vi "Uframe-LVDT_Cal.vi"() -> ()   [LabVIEW 2010]
uses:
  <vilib>/Platform/TimedLoop/XDataNode/XDataNode.xnode
  <vilib>/Platform/TimedLoop/XDataNode/timing_clust.ctl
  <vilib>/Platform/TimedLoop/XDataNode/nitl_modes.ctl
  <vilib>/Platform/TimedLoop/XDataNode/wakeup.ctl
  <vilib>/Platform/TimedLoop/XDataNode/XDNodeRunTimeDep.lvlib
panel:
  out "Numeric":i32
  in  "Displacement (inch)":dbl min=-1.0 max=60.0 step=0.01
  in  "Begin":bool
  in  "Stop":bool
  out "Disp Vs Time":cluster{dbl[], dbl[]}(graph)={[-724.1250113144533, -724.195323815552, -724.2656363166506, -724.3359488177492, -724.4062613188479, -724.4765738199465, -724.5468863210451, -724.6171988221438, -724.7461050741579, -724.9218863269045, -725.0976675796511, -725.2851675825808, -725.4492300851442], [-11.89350874713131, -11.896152101474941, -11.894229661847117, -11.89350874707076, -11.890865392620372, -11.895671491596438, -11.895911796524977, -11.899756675680168, -11.899035760801853, -11.90552399441818, -11.907927043887174, -11.905283689458143, -11.914655582386047]}
  in  "File Name":string="Test"
  in  "File Path":path=path "C:/cygwin/home/Smarter Materials/Users 2010_2011/Chris_Montgomery"
  in  "Sample Notes":string
  in  "Data Acquisition Interval (s)":dbl min=0.01 max=60.0 step=0.01
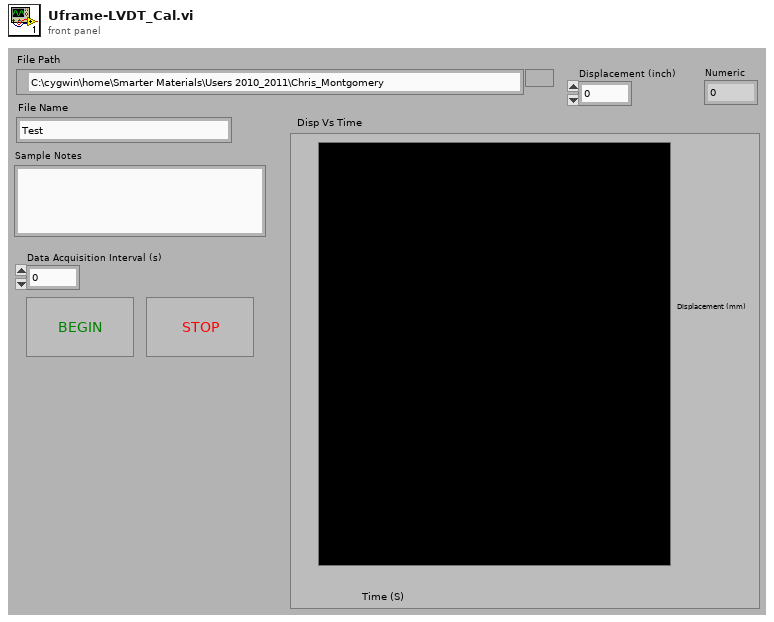
[diagram p1: front panel]
types:
  T1 = typedef "XDNodeRunTimeDep.lvlib/timing_clust.ctl" = cluster{"Expected End [f-1]":u64, "Actual End [f-1]":u64, "Finished Late? [f-1]":bool, "Expected End [i-1]":u64, "Actual End [i-1]":u64, "Finished Late? [i-1]":bool, "Expected Start [i]":u64, "Actual Start [i]":u64, "Expected Start [f]":u64, "Actual Start [f]":u64, "Source Name":string, "Structure Name":string, "Period":i64, "Deadline":i64, "Offset":i64, "Start":i64, "Priority":i32, "Timeout":i32, "Mode":T2, "Wakeup Reason":T3, "Error":errorcluster, "Source Type":string, "Secondary Source Type":string, "Global End Time":u64, "Global Start Time":u64, "Frame Duration":u64, "Iteration Duration":u64, "Assigned CPU":i32, "I/O Scan Engine Mode":u32}
  T2 = typedef "XDNodeRunTimeDep.lvlib/nitl_modes.ctl" = enum32{"No Change", "Process missed periods, maintain original phase", "Discard missed periods, maintain original phase", "Process missed periods, ignore original phase", "Discard missed periods, ignore original phase"}
  T3 = typedef "XDNodeRunTimeDep.lvlib/wakeup.ctl" = enum32{"Normal", "Aborted", "Asynchronous wakeup", "Timing source error", "Timed loop error", "Timeout"}
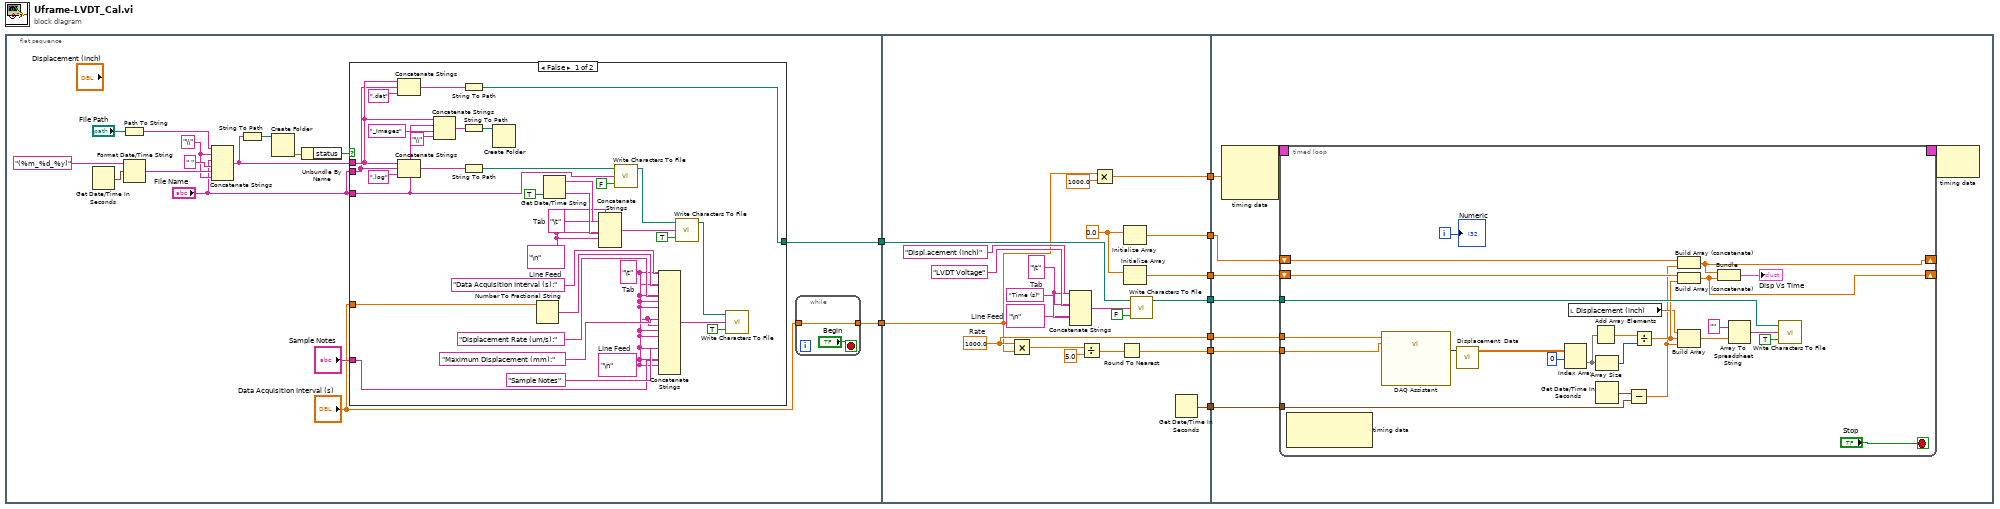
[diagram p0: block diagram]
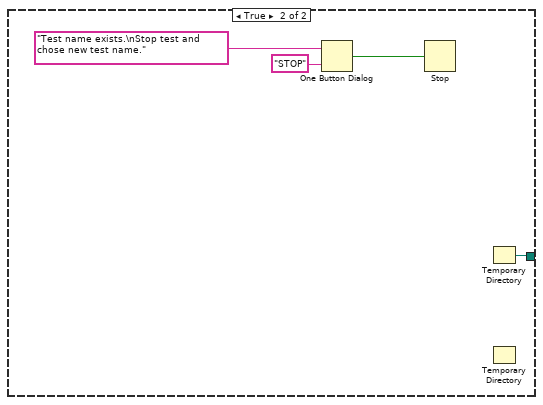
[diagram p2: hidden frame]
diagram:
  n1 = flat-sequence {
    tunnel: [w12] -> w2
    tunnel: [w11] -> w1
    tunnel: [w81] -> w9
    tunnel: [w80] -> w8
    tunnel: [w79] -> w7
    tunnel: [w78] -> w6
    tunnel: [w77] -> w5
    tunnel: [w76] -> w4
    tunnel: [w70] -> w3
    tunnel: w2 -> [w69]
    tunnel: w1 -> [w68]
    tunnel: w9 -> [w93]
    tunnel: w8 -> [w92]
    tunnel: w7 -> [w91]
    tunnel: w6 -> [w90]
    tunnel: w5 -> [w89]
    tunnel: w4 -> [w88]
    tunnel: w3 -> [w87]
    frame #0 {
      w19 = "\\"
      n2 = Get Date/Time In Seconds() -> (seconds since 1Jan1904=w22:timestamp)
      n3 = Path To String(path="File Path") -> (string=w25:string)
      n4 = Format Date/Time String(time format string (%c)="(%m_%d_%y)", seconds (now)=w22) -> (date/time string=w21:string)  [unwired: 1 in]
      n5 = Concatenate Strings(w25, w19, "File Name", " ", w21, w19) -> (w14:string)
      n6 = String To Path(string=w14) -> (path=w18:path)
      n7 = Create Folder(path (use dialog)=w18) -> (error out=w24:errorcluster)  [unwired: 2 in, 2 out]
      n8 = Unbundle By Name(w24) -> ("status"=w17:bool)
      n9 = case shown="False" w17 {
        tunnel: w14 -> [w30 _]
        tunnel: "File Name" -> [w29 _]
        tunnel: "File Name" -> [w34 _]
        tunnel: "Data Acquisition Interval (s)" -> [w49 _]
        tunnel: "Sample Notes" -> [w36 _]
        tunnel: [w31 w62] -> w12
        frame False {
          w28 = "\t"  # Tab
          w35 = "\n"  # Line Feed
          w52 = "\t"  # Tab
          w46 = "\n"  # Line Feed
          n10 = Concatenate Strings(w30, w29, ".dat") -> (w32:string)
          n11 = Concatenate Strings(w30, w29, ".log") -> (w54:string)
          n12 = Concatenate Strings(w30, w34, "_Images", "\\") -> (w42:string)
          n13 = String To Path(string=w32) -> (path=w31:path)
          n14 = String To Path(string=w42) -> (path=w41:path)
          n15 = String To Path(string=w54) -> (path=w59:path)
          n16 = Create Folder(path (use dialog)=w41) -> ()  [unwired: 2 in, 3 out]
          n17 = Number To Fractional String(number=w49) -> (F-format string=w40:string)  [unwired: 3 in]
          n18 = Get Date/Time String(want seconds? (F)=TRUE) -> (date string=w57:string, time string=w56:string)  [unwired: 2 in]
          n19 = Concatenate Strings(w46, w57, w52, w56, w46, w46) -> (w58:string)
          n20 = call <vilib>:"Write Characters To File.vi"("append to file? (new file:F)"=FALSE, "character string"=w34, "file path (dialog if empty)"=w59) -> ("new file path (Not A Path if cancelled)"=w55:path)  [unwired: 2 in]
          n21 = Concatenate Strings("Data Acquisition Interval (s):", w28, w40, w35, "Displacement Rate (um/s):", w28, w28, w35, "Maximum Displacement (mm):", w28, w28, w35, w35, "Sample Notes", w35, w36, w35, w35) -> (w47:string)
          n22 = call <vilib>:"Write Characters To File.vi"("append to file? (new file:F)"=TRUE, "character string"=w58, "file path (dialog if empty)"=w55) -> ("new file path (Not A Path if cancelled)"=w50:path)  [unwired: 2 in]
          n23 = call <vilib>:"Write Characters To File.vi"("append to file? (new file:F)"=TRUE, "character string"=w47, "file path (dialog if empty)"=w50) -> ()  [unwired: 2 in, 1 out]
        }
        frame True {
          n24 = One Button Dialog(message="Test name exists.\nStop test and chose new test name.", button name ("OK")="STOP") -> (true=w63:bool)
          n25 = Stop(stop? (T)=w63) -> ()
          n26 = Temporary Directory() -> (w62:path)
          n27 = Temporary Directory() -> ()  [unwired: 1 out]
        }
      }
      n28 = while {
        tunnel: [w26] -> w11
        tunnel: "Data Acquisition Interval (s)" -> [w26]
        stop <- "Begin" stop-if-true
      }
    }
    frame #1 {
      w66 = "\n"  # Line Feed
      w71 = "\t"  # Tab
      w78 = 1000.0  # Rate
      w85 = 0.0
      n29 = Multiply(x=w78, y=w68) -> (x*y=w84:dbl)
      n30 = Concatenate Strings("Displ.acement (inch)", w71, "LVDT Voltage" ("Substring"), w71, "Time (s)" ("string"), w66) -> (w74:string)
      n31 = Divide(x=w84, y=5.0) -> (x/y=w82:dbl)
      n32 = Multiply(x=w68, y=1000.0) -> (x*y=w81:dbl)
      n33 = Round To Nearest(number=w82) -> (nearest integer value=w77:dbl)
      n34 = Initialize Array(w85) -> (w79:dbl[])  [unwired: 1 in]
      n35 = Initialize Array(w85) -> (w80:dbl[])  [unwired: 1 in]
      n36 = call <vilib>:"Write Characters To File.vi"("append to file? (new file:F)"=FALSE, "character string"=w74, "file path (dialog if empty)"=w69) -> ("new file path (Not A Path if cancelled)"=w70:path)  [unwired: 2 in]
      n37 = Get Date/Time In Seconds() -> (seconds since 1Jan1904=w76:timestamp)
    }
    frame #2 {
      n38 = node-c288 ("Input Node")(w93) -> (w95:T1)  [unwired: 2 in]
      n39 = timed-loop {
        shift-left: w92 -> [w105]
        shift-right: [w96] -> _
        shift-left: w91 -> [w106]
        shift-right: [w97] -> _
        timing-out: [_] -> w94
        timing: w95 -> [_]
        tunnel: w89 -> [w110]
        tunnel: w90 -> [w109]
        tunnel: w88 -> [w104]
        tunnel: w87 -> [w103]
        i -> [w100]
        stop <- "Stop" stop-if-true
        n40 = node-c288() -> ()  [unwired: 1 in, 2 out]
        n41 = call "DAQ Assistant"("rate"=w109, "number of samples"=w110) -> ("data"=w108:dynamicdata)  [unwired: 15 in, 2 out]
        n42 = call "Displacement  Data"("Dynamic Data Type"=w108) -> ("Array"=w115:dbl[][])  [unwired: 3 in]
        n43 = Index Array(array=w115, index (row)=0) -> (element=w113:dbl[])  [unwired: 1 in]
        n44 = local read "Displacement (inch)"() -> (w101:dbl)
        n45 = Add Array Elements(numeric array=w113) -> (sum=w112:dbl)
        n46 = Array Size(array=w113) -> (size(s)=w111:i32)
        n47 = Get Date/Time In Seconds() -> (seconds since 1Jan1904=w114:timestamp)
        n48 = Subtract(x=w114, y=w104) -> (x-y=w99:dbl)
        n49 = Divide(x=w112, y=w111) -> (x/y=w102:dbl)
        n50 = Build Array (concatenate)(w106, w99) -> (w97:dbl[])
        n51 = Build Array (concatenate)(w105, w102) -> (w96:dbl[])
        n52 = Build Array(w101, w102, w99) -> (w117:dbl[])
        n53 = Bundle(w97, w96) -> (→"Disp Vs Time":cluster{dbl[], dbl[]})  [unwired: 1 in]
        n54 = Array To Spreadsheet String(array=w117, 3:"" ("format string")) -> (spreadsheet string=w119:string)  [unwired: 1 in]
        n55 = call <vilib>:"Write Characters To File.vi"("append to file? (new file:F)"=TRUE, "character string"=w119, "file path (dialog if empty)"=w103) -> ()  [unwired: 2 in, 1 out]
        "Numeric" <- w100
      }
      n56 = node-c288(w94) -> ()  [unwired: 1 out]
    }
  }
